vi "Roll.vi"(8 "error in (no error)":errorcluster, 11 "Dice in":refnum<class "Dice.lvclass">) -> (0 "error out":errorcluster, 3 "Dice out":refnum<class "Dice.lvclass">)   [LabVIEW 2016, in "Dice.lvclass"]
uses:
  Dice.lvclass
  Dice.lvclass/Dice.ctl
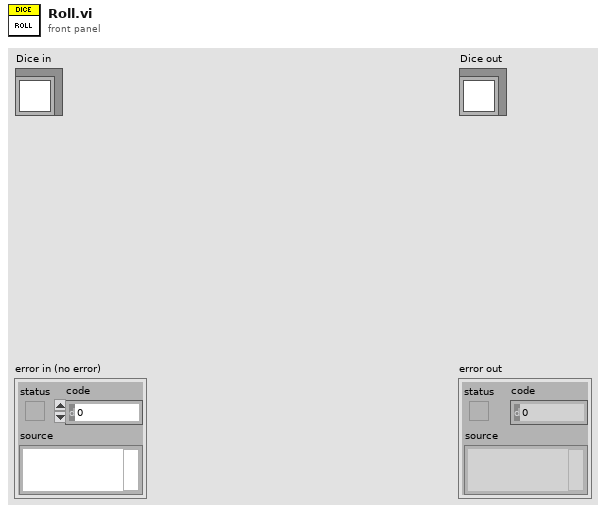
[diagram p1: front panel]
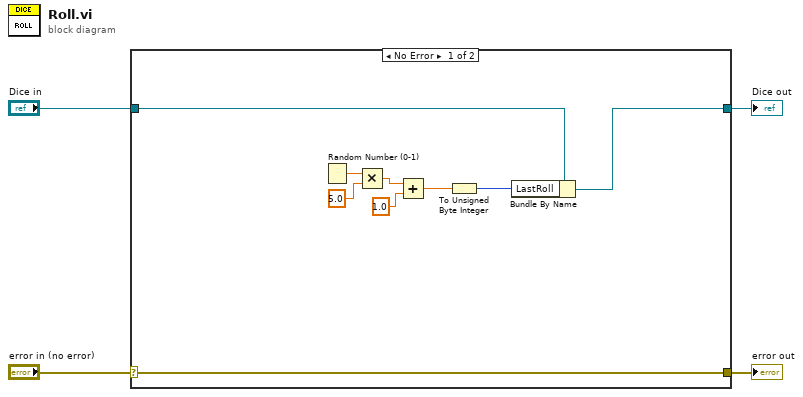
[diagram p0: block diagram]
diagram:
  n1 = case shown="No Error" "error in (no error)" {
    selector: "error in (no error)" -> [w13 w15]
    tunnel: [w13 w15] -> w3
    tunnel: [w11 w14] -> w1
    tunnel: "Dice in" -> [w12 w14]
    frame No Error {
      n2 = Random Number (0-1)() -> (number: 0 to 1=w10:dbl)
      n3 = Multiply(x=w10, y=5.0) -> (x*y=w8:dbl)
      n4 = Add(x=w8, y=1.0) -> (x+y=w6:dbl)
      n5 = To Unsigned Byte Integer(number=w6) -> (unsigned 8bit integer=w5:u8)
      n6 = Bundle By Name(cluster=w12, "LastRoll"=w5) -> (w11:refnum<class "Dice.lvclass">)
    }
    frame Error {
    }
  }
  "error out" <- w3
  "Dice out" <- w1
